vi "Get Values.vi"() -> (0 "Bottom Float Switch":bool, 1 "Top Float Switch":bool, 2 "Water level":i32(slide) scale=0.0..300.0)   [LabVIEW 2013]
uses:
  Water Tank Global.vi
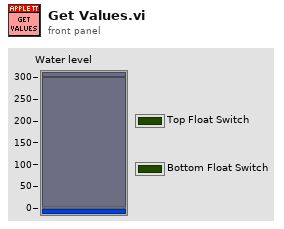
[diagram p1: front panel]
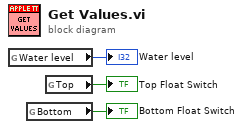
[diagram p0: block diagram]
diagram:
  n1 = global read "Water Tank Global.vi" "Water level"() -> (→"Water level":i32)
  n2 = global read "Water Tank Global.vi" "Bottom"() -> (→"Bottom Float Switch":bool)
  n3 = global read "Water Tank Global.vi" "Top"() -> (→"Top Float Switch":bool)
